vi "Array Get Size.vi"(8 "error in (no error)":errorcluster, 11 "Array DVR in":refnum<data-value>) -> (0 "error out":errorcluster, 2 "Size":i32, 3 "Array DVR out":refnum<data-value>)   [LabVIEW 2012, in "MDSplus.lvlib"]
uses:
  <vilib>/MDSplus/Library/MDSplus.lvlib
  <vilib>/MDSplus/Classes/Data_Class/Array_Class/Array.lvclass
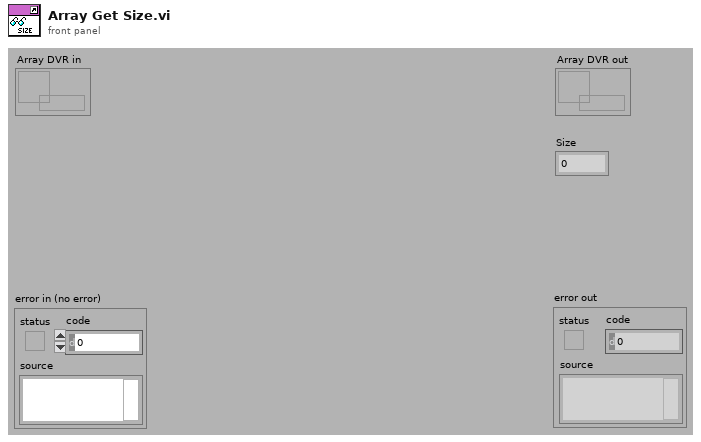
[diagram p1: front panel]
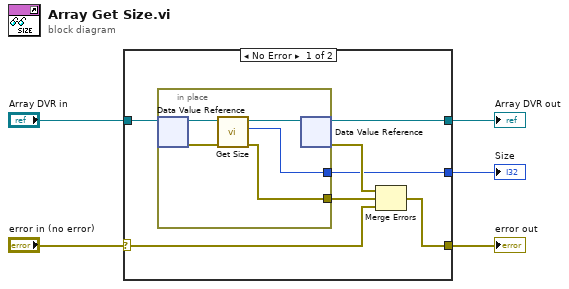
[diagram p0: block diagram]
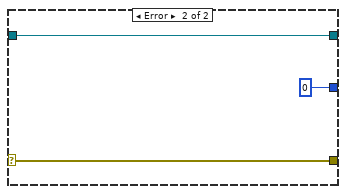
[diagram p2: hidden frame]
diagram:
  n1 = case shown="No Error" "error in (no error)" {
    selector: "error in (no error)" -> [w10 w20]
    tunnel: "Array DVR in" -> [w12 w19]
    tunnel: [w8 w20] -> w5
    tunnel: [w7 w19] -> w2
    tunnel: [w6 0 ("SGL array out")] -> w1
    frame No Error {
      n2 = in-place {
        in-place-border: [w15] -> w11
        in-place-border: [w13] -> w6
        n3 = in-place-dvr #1(w12) -> (w17:refnum<class "Array.lvclass">, w14:errorcluster)
        n4 = call-dynamic "Get Size.vi"("error in (no error)"=w14, "Array in"=w17) -> ("error out"=w15:errorcluster, "Size out"=w13:i32, "Array out"=w16:refnum<class "Array.lvclass">)  [unwired: 7 in]
        n5 = in-place-dvr #1(w16) -> (w7:refnum<data-value>, w9:errorcluster)
      }
      n6 = Merge Errors(w9, w11, w10) -> (w8:errorcluster)
    }
    frame Error {
    }
  }
  "error out" <- w5
  "Array DVR out" <- w2
  "Size" <- w1
